vi "odor config error (sub-vi).vi"() -> (0 "error":errorcluster)   [LabVIEW 2021]
uses:
  type-defs/project_custom_error_codes_ring (type def).ctl
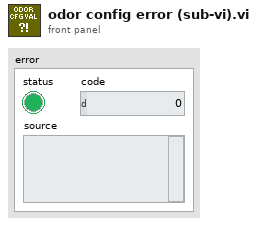
[diagram p1: front panel]
types:
  T1 = typedef "project_custom_error_codes_ring (type def).ctl" = i32
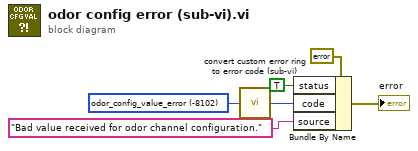
[diagram p0: block diagram]
diagram:
  w4 = T1 -8102 items=["parse_failure"=-8001, "arduino_failure"=-8002, "manifold_config_value_error"=-8101, "odor_config_value_error"=-8102] ("Ring")
  n1 = call "convert custom error ring to error code (sub-vi).vi"("custom error ring"=w4) -> ("error code"=w3:i32)  [unwired: 4 in]
  n2 = Bundle By Name(cluster=errorcluster {"status"=FALSE, "code"=0, "source"=""} ("error constant"), "status"=TRUE, "code"=w3, "source"="Bad value received for odor channel configuration.") -> (→"error":errorcluster)
